vi "SELECIONA STRING DA APLICACAO.vi"() -> ()   [LabVIEW 2019]
panel:
  out "Array":string[](array[string])
  in  "SALVAR":bool
  in  "FRA":bool
  in  "FLO":bool
  in  "RAN":bool
  in  "NUM":bool
  # "NUM"
  # "RAN"
  # "FRA"
  # "FLO"
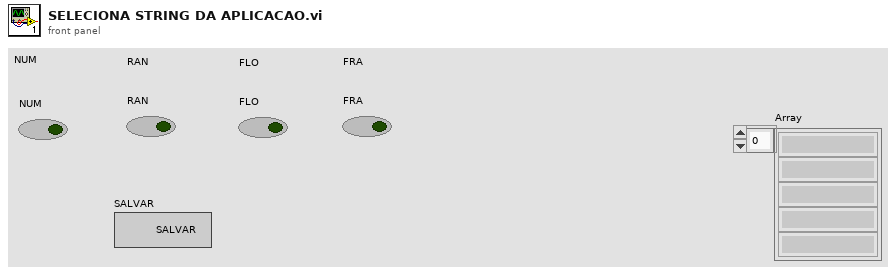
[diagram p1: front panel]
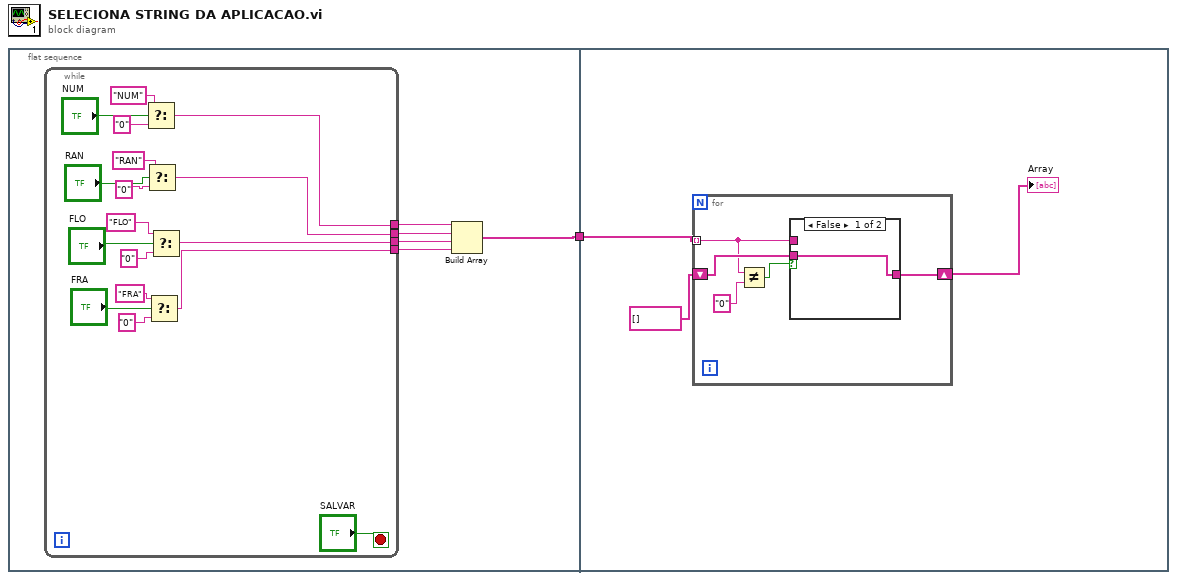
[diagram p0: block diagram]
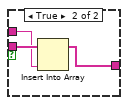
[diagram p2: hidden frame]
diagram:
  n1 = flat-sequence {
    tunnel: [w2] -> w1
    tunnel: w1 -> [w26]
    frame #0 {
      n2 = while {
        tunnel: [w11] -> w6
        tunnel: [w10] -> w5
        tunnel: [w9] -> w4
        tunnel: [w8] -> w3
        stop <- "SALVAR" stop-if-true
        n3 = Select(t="NUM", s="NUM", f="0") -> (s? t:f=w11:string)
        n4 = Select(t="RAN", s="RAN", f="0") -> (s? t:f=w10:string)
        n5 = Select(t="FRA", s="FRA", f="0") -> (s? t:f=w8:string)
        n6 = Select(t="FLO", s="FLO", f="0") -> (s? t:f=w9:string)
      }
      n7 = Build Array(w6, w5, w4, w3) -> (w2:string[])
    }
    frame #1 {
      n8 = for {
        tunnel: w26 -> [w27] mode=indexing
        shift-right: [w30] -> w24
        shift-left: string[] [] ("Array") -> [w31]
        n9 = Not Equal?(x=w27, y="0") -> (x != y?=w28:bool)
        n10 = case shown="False" w28 {
          tunnel: w31 -> [w32 w35]
          tunnel: [w32 w34] -> w30
          tunnel: w27 -> [_ w33]
          frame False {
          }
          frame True {
            n11 = Insert Into Array(array=w35, new element=w33) -> (w34:string[])  [unwired: 1 in]
          }
        }
      }
      "Array" <- w24
    }
  }
